vi "New Line from Data.vi"(0 "Mode":string, 1 "DAQ A":dbl, 2 "Setting":dbl, 3 "DAQ R":dbl, 4 "BK V":dbl, 6 "DateTime Stamp":timestamp, 7 "BK I":dbl, 8 "ID":string, 9 "BK R":dbl, 10 "Delimiter Character":string, 11 "BK P":dbl, 13 "DAQ T":dbl) -> (14 "String":string)   [LabVIEW 2010]
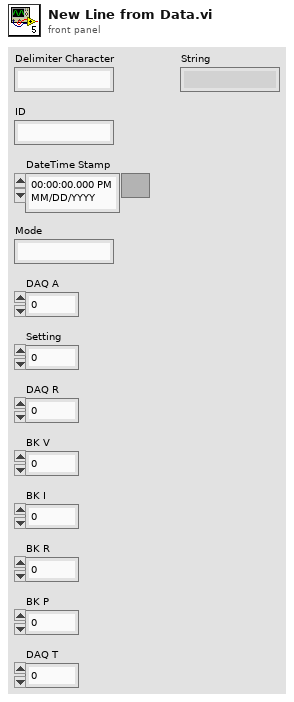
[diagram p1: front panel]
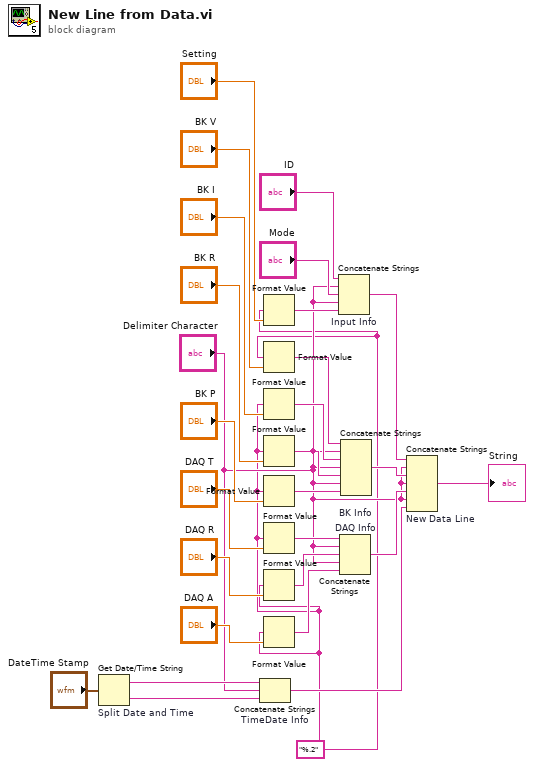
[diagram p0: block diagram]
diagram:
  w1 = "%.2"
  n1 = Get Date/Time String "Split Date and Time"(seconds (now)="DateTime Stamp") -> (date string=w9:string, time string=w10:string)  [unwired: 2 in]
  n2 = Concatenate Strings "TimeDate Info"(w9, "Delimiter Character", w10) -> (w6:string)
  n3 = Format Value(format string=w1, value (0)="Setting") -> (output string=w28:string)  [unwired: 1 in]
  n4 = Format Value(format string=w1, value (0)="BK V") -> (output string=w21:string)  [unwired: 1 in]
  n5 = Format Value(format string=w1, value (0)="BK I") -> (output string=w22:string)  [unwired: 1 in]
  n6 = Format Value(format string=w1, value (0)="BK R") -> (output string=w23:string)  [unwired: 1 in]
  n7 = Format Value(format string=w1, value (0)="BK P") -> (output string=w24:string)  [unwired: 1 in]
  n8 = Format Value(format string=w1, value (0)="DAQ T") -> (output string=w18:string)  [unwired: 1 in]
  n9 = Format Value(format string=w1, value (0)="DAQ R") -> (output string=w19:string)  [unwired: 1 in]
  n10 = Format Value(format string=w1, value (0)="DAQ A") -> (output string=w20:string)  [unwired: 1 in]
  n11 = Concatenate Strings "Input Info"("ID", "Delimiter Character", "Mode", "Delimiter Character", w28) -> (w3:string)
  n12 = Concatenate Strings "DAQ Info"(w18, "Delimiter Character", w19, "Delimiter Character", w20) -> (w5:string)
  n13 = Concatenate Strings "BK Info"(w21, "Delimiter Character", w22, "Delimiter Character", w23, "Delimiter Character", w24) -> (w4:string)
  n14 = Concatenate Strings "New Data Line"(w3, "Delimiter Character", w4, "Delimiter Character", w5, "Delimiter Character", w6) -> (→"String":string)
